vi "RSZVB Read Time Samples Data.vi"(8 "error in (no error)":errorcluster {"code" format="%.0x"}, 10 "Channel (Trace) (1)":i32=1, 11 "VISA session":refnum<visa-resource-name>) -> (0 "error out":errorcluster {"code" format="%.0x"}, 3 "dup VISA session":refnum<visa-resource-name>, 5 "Trace Data":dbl[](array[numeric]) format="%^.3e")   [LabVIEW 2011]
doc: "This VI reads the SSRAM Data in Pulse Profile Mode. Only for traces with wave quantities (a- or b- waves)\n\nRemote-control command(s):\nFORMat[:DATA] REAL ,32\nCALCulate<Ch>:DATA? TSData"
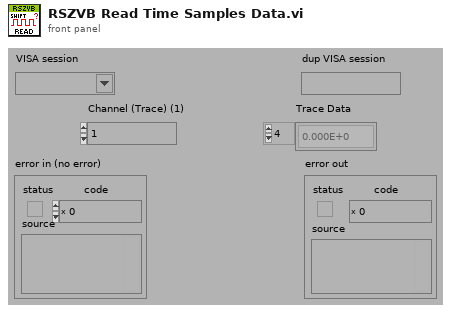
[diagram p1: front panel]
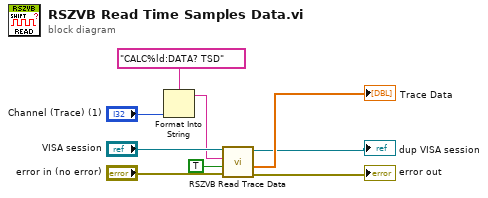
[diagram p0: block diagram]
diagram:
  n1 = Format Into String(format string="CALC%ld:DATA? TSD", "Channel (Trace) (1)") -> (resulting string=w5:string)  [unwired: 2 in, 1 out]
  n2 = call "RSZVB Read Trace Data.vi"("error in (no error)"="error in (no error)", "Force ASCII"=TRUE, "Buffer"=w5, "VISA session"="VISA session") -> ("error out"=→"error out":errorcluster, "Trace Data"=→"Trace Data":dbl[], "dup VISA session"=→"dup VISA session":refnum<visa-resource-name>)  [unwired: 5 in]
